vi "Match_MAC.vi"(7 "MAC & Name In":string[][](array[string]), 8 "Error In":errorcluster, 11 "Network Map In":string) -> (0 "Error Out":errorcluster, 3 "Drfiter IP Addresses Out":string[][](array[string]))   [LabVIEW 2017]
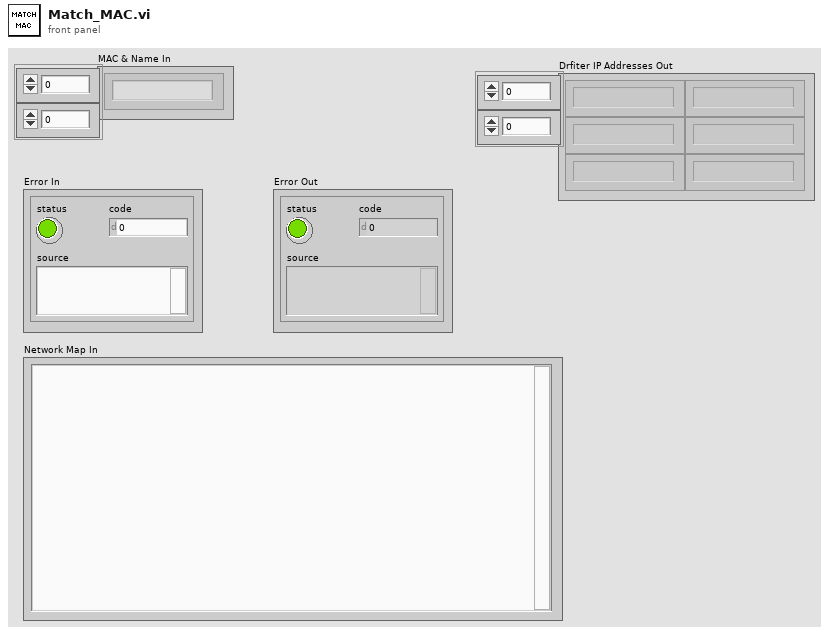
[diagram p1: front panel]
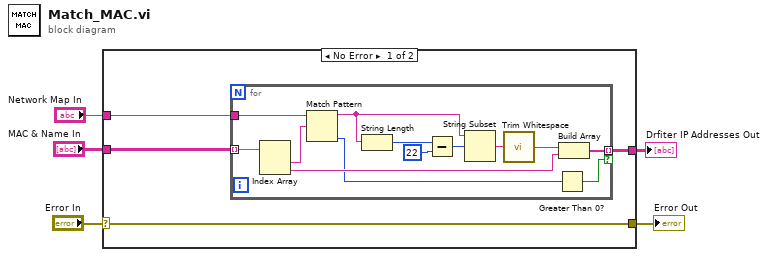
[diagram p0: block diagram]
diagram:
  n1 = case shown="No Error" "Error In" {
    selector: "Error In" -> [w8 w23]
    tunnel: [w9 _] -> w1
    tunnel: "MAC & Name In" -> [w6 _]
    tunnel: [w8 w23] -> w4
    tunnel: "Network Map In" -> [w7 _]
    frame No Error {
      n2 = for {
        tunnel: [w17] -> w9 mode=indexing if=w13
        tunnel: w7 -> [w18]
        tunnel: w6 -> [w16] mode=indexing
        n3 = Index Array(array=w16) -> (element #1=w15:string, element #2=w14:string)  [unwired: 2 in]
        n4 = Match Pattern(string=w18, regular expression=w15) -> (before substring=w22:string, offset past match=w12:i32)  [unwired: 1 in, 2 out]
        n5 = String Length(string=w22) -> (length=w21:i32)
        n6 = Subtract(x=w21, y=22) -> (x-y=w20:i32)
        n7 = String Subset(string=w22, offset (0)=w20) -> (substring=w11:string)  [unwired: 1 in]
        n8 = call <vilib>:"Trim Whitespace.vi"("string"=w11) -> ("trimmed string"=w10:string)  [unwired: 1 in]
        n9 = Greater Than 0?(x=w12) -> (x > 0?=w13:bool)
        n10 = Build Array(w10, w14) -> (w17:string[])
      }
    }
    frame Error {
    }
  }
  "Error Out" <- w4
  "Drfiter IP Addresses Out" <- w1
